vi "ics_ids_save_2D_Analog_PMT.vi"(0 "pixels":i32, 1 "filename":string, 3 "folder":path=path "D:/User/Sergey/ids_ics_trainer", 5 "Dwell":dbl, 7 "data":dbl[][](array[numeric]), 9 "Range":dbl, 11 "error in":errorcluster) -> (4 "saved":bool, 15 "error out":errorcluster)   [LabVIEW 2009]
panel:
  out "output array":dbl[](array[numeric])
  out "text":string
  in  "scale I":i32=1
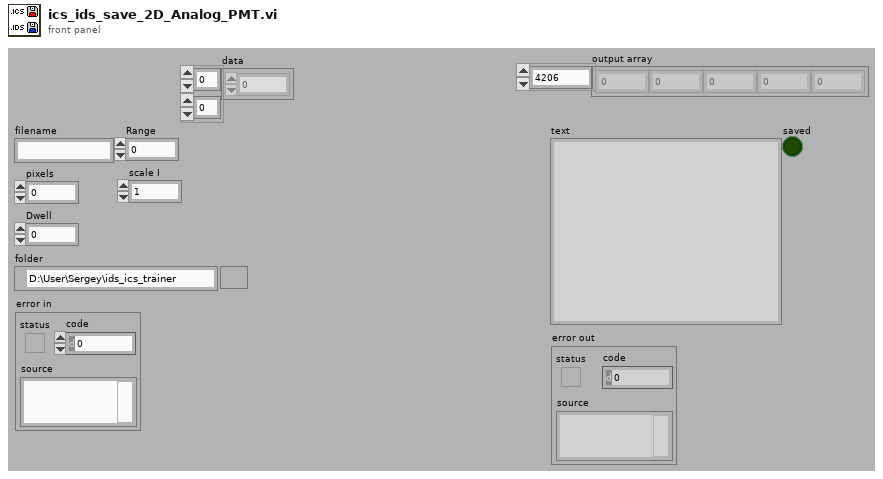
[diagram p1: front panel]
types:
  T1 = enum16{"open", "replace", "create", "open or create", "replace or create", "replace or create with confirmation"}
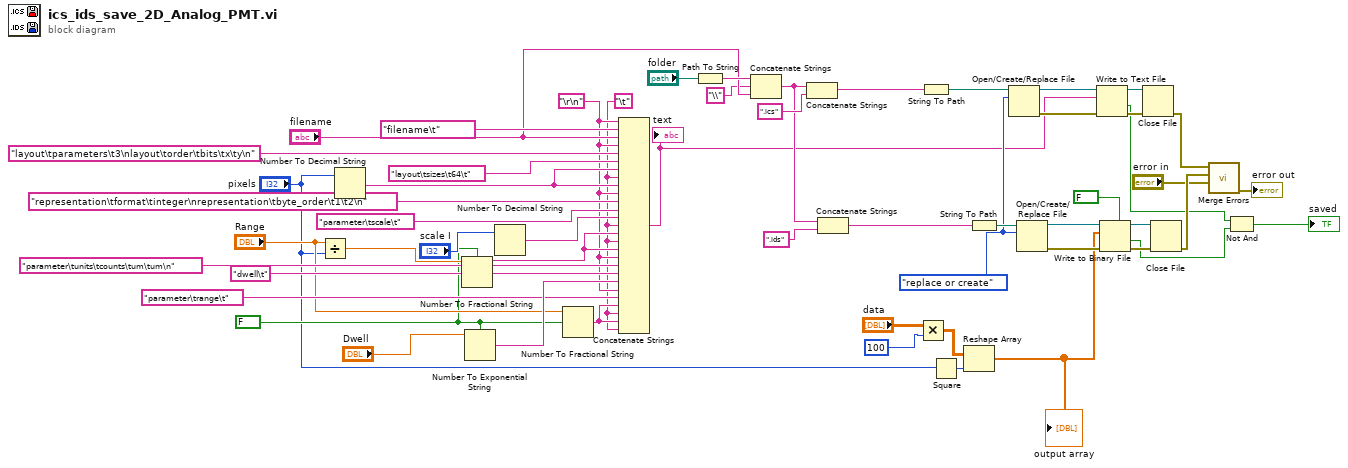
[diagram p0: block diagram]
diagram:
  w12 = FALSE ("use system decimal point (T)")
  w31 = T1."replace or create" ("operation (0:open)")
  w13 = "\t"
  w33 = "\r\n"
  n1 = Divide(x="Range", y="pixels") -> (x/y=w48:dbl)
  n2 = Number To Decimal String(number="pixels") -> (decimal integer string=w53:string)  [unwired: 1 in]
  n3 = Number To Fractional String(use system decimal point (T)=w12, number=w48) -> (F-format string=w47:string)  [unwired: 2 in]
  n4 = Number To Exponential String(number="Dwell", 1:w12) -> (E-format string=w42:string)  [unwired: 2 in]
  n5 = Number To Decimal String(number="scale I") -> (decimal integer string=w49:string)  [unwired: 1 in]
  n6 = Number To Fractional String(use system decimal point (T)=w12, number="Range") -> (F-format string=w14:string)  [unwired: 2 in]
  n7 = Concatenate Strings(w33, "filename\t" ("string"), "filename", w33, "layout\tparameters\t3\nlayout\torder\tbits\tx\ty\n" ("string"), "layout\tsizes\t64\t" ("string"), w53, w13, w53, w33, "representation\tformat\tinteger\nrepresentation\tbyte_order\t1\t2\n" ("string"), "parameter\tscale\t" ("string"), w49, w13, w47, w13, w47, w33, "parameter\tunits\tcounts\tum\tum\n" ("string"), "dwell\t" ("string"), w42, w33, "parameter\trange\t" ("string"), w14, w13, w14, w13) -> (w24:string)
  "text" <- w24
  n8 = Path To String(path="folder") -> (string=w37:string)
  n9 = Concatenate Strings(w37, "\\" ("string"), "filename") -> (w26:string)
  n10 = Concatenate Strings(w26, ".ics" ("string")) -> (w28:string)
  n11 = Concatenate Strings(w26, ".ids" ("string")) -> (w25:string)
  n12 = Multiply(x="data", y=100) -> (x*y=w2:dbl[][])
  n13 = String To Path(string=w28) -> (path=w35:path)
  n14 = Square(x="pixels") -> (x^2=w18:i32)
  n15 = Reshape Array(w2, w18) -> (w17:dbl[])
  "output array" <- w17
  n16 = String To Path(string=w25) -> (path=w32:path)
  n17 = Open/Create/Replace File(file path (use dialog)=w35, operation (0:open)=w31) -> (refnum out=w39:refnum<file>, error out=w38:errorcluster)  [unwired: 4 in, 1 out]
  n18 = Open/Create/Replace File(file path (use dialog)=w32, operation (0:open)=w31) -> (refnum out=w21:refnum<file>, error out=w20:errorcluster)  [unwired: 4 in, 1 out]
  n19 = Write to Text File(file (use dialog)=w39, text=w24, error in=w38) -> (refnum out=w41:refnum<file>, cancelled=w7:bool, error out=w40:errorcluster)  [unwired: 1 in]
  n20 = Write to Binary File(file (use dialog)=w21, data=w17, error in=w20, 5:FALSE ("prepend array or string size? (T)")) -> (refnum out=w22:refnum<file>, cancelled=w6:bool, error out=w23:errorcluster)  [unwired: 2 in]
  n21 = Close File(refnum=w41, error in=w40) -> (error out=w11:errorcluster)  [unwired: 1 out]
  n22 = Close File(refnum=w22, error in=w23) -> (error out=w10:errorcluster)  [unwired: 1 out]
  n23 = call <vilib>:"Merge Errors.vi"("error in 3 (no error)"="error in", "error in 2 (no error)"=w10, "error in 1 (no error)"=w11) -> ("error out"=→"error out":errorcluster)  [unwired: 4 in]
  n24 = Not And(1:w6, 2:w7) -> (0:→"saved":bool)
